vi "Initialize.vi"(8 "error in (no error)":errorcluster, 9 "Reset (True)":bool=TRUE, 10 "ID Query (True)":bool=TRUE, 11 "VISA resource name":refnum<visa-resource-name>) -> (0 "error out":errorcluster, 3 "VISA resource name out":refnum<visa-resource-name>)   [LabVIEW 2024, in "U1250 Series Digital Multimeter.lvlib"]
doc: "Establishes communication with the instrument and optionally performs an instrument identification query and/or an instrument reset. It also places the instrument in a default state needed for other instrument driver operations. Therefore, call this VI before calling other instrument driver VIs for this instrument. Generally, you need to call the <b>Initialize</b> VI only once at the beginning of an application."
uses:
  U1250 Series Digital Multimeter.lvlib
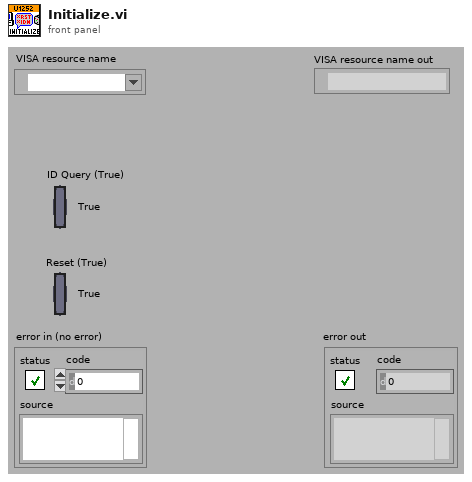
[diagram p1: front panel]
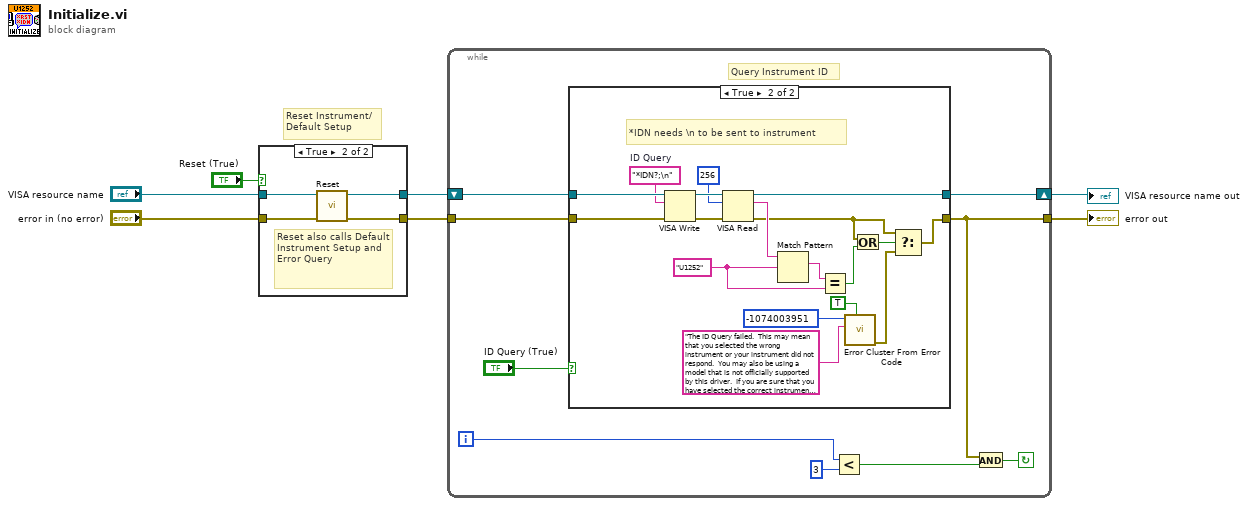
[diagram p0: block diagram]
diagram:
  # "Reset Instrument/\nDefault Setup"
  n1 = case shown="True" "Reset (True)" {
    tunnel: "error in (no error)" -> [w8 w10]
    tunnel: [w8 w13] -> w5
    tunnel: "VISA resource name" -> [w9 w11]
    tunnel: [w9 w12] -> w6
    frame False {
    }
    frame True {
      # "Reset also calls Default Instrument Setup and Error Query"
      n2 = call "Reset.vi"("error in (no error)"=w10, "VISA resource name"=w11) -> ("error out"=w13:errorcluster, "VISA resource name out"=w12:refnum<visa-resource-name>)  [unwired: 8 in]
    }
  }
  n3 = while {
    shift-right: [w19] -> w2
    shift-left: w6 -> [w21]
    tunnel: w5 -> [w20]
    tunnel: [w17] -> w1
    i -> [w16]
    stop <- w18 continue-if-true
    # "Query Instrument ID"
    n4 = case shown="True" "ID Query (True)" {
      tunnel: [w23 w42] -> w17
      tunnel: [w24 w39] -> w19
      tunnel: w21 -> [w24 w40]
      tunnel: w20 -> [w23 w41]
      frame False {
      }
      frame True {
        w34 = "*IDN?;\n"  # ID Query
        w27 = "U1252"
        # "*IDN needs \\n to be sent to instrument"
        n5 = VISA Write(VISA resource name=w40, write buffer=w34, error in (no error)=w41) -> (VISA resource name out=w37:refnum<visa-resource-name>, error out=w36:errorcluster)  [unwired: 1 out]
        n6 = VISA Read(VISA resource name=w37, byte count=u32 256, error in (no error)=w36) -> (VISA resource name out=w39:refnum<visa-resource-name>, read buffer=w38:string, error out=w25:errorcluster)  [unwired: 1 out]
        n7 = Match Pattern(string=w38, regular expression=w27) -> (match substring=w28:string)  [unwired: 1 in, 3 out]
        n8 = Equal?(x=w28, y=w27) -> (x = y?=w26:bool)
        n9 = call <vilib>:"Error Cluster From Error Code.vi"("show call chain? (False)"=TRUE, "error message (\"\")"="The ID Query failed.  This may mean that you selected the wrong instrument or your instrument did not respond.  You may also be using a model that is not officially supported by this driver.  If you are sure that you have selected the correct instrument and it is responding, try disabling the ID Query." ("Source (VI Name)"), "error code (0)"=-1074003951 ("Code")) -> ("error out"=w33:errorcluster)  [unwired: 6 in]
        n10 = Or(x=w25, y=w26) -> (x .or. y?=w29:bool)
        n11 = Select(t=w25, s=w29, f=w33) -> (s? t:f=w42:errorcluster)
      }
    }
    n12 = Less?(x=w16, y=3) -> (x < y?=w14:bool)
    n13 = And(x=w17, y=w14) -> (x .and. y?=w18:bool)
  }
  "VISA resource name out" <- w2
  "error out" <- w1
